vi "AddSingleOperation.vi"(6 "Timeout in ms (-1)":i32, 7 "At opposite end?":bool, 8 "error in (no error)":errorcluster, 10 "Operation":T1, 11 "SMP in":refnum<class "SMP.lvclass">) -> (0 "error out":errorcluster, 3 "SMP out":refnum<class "SMP.lvclass">)   [LabVIEW 2013, in "SMP.lvclass"]
doc: "Adds one individual operation, to the internal operations queue of the SMP object.\n\n<b>At opposite end?: </b>Set to TRUE to add the operation to the front of the internal operations queue. Default is FALSE.\n\n<b>Operations: </b>The operations to be added. Each operation has a name and data associated with it. Use this Data field to provide any data that the operation needs, except data produced by the operation which executes before it.\n\n<b>Timeout: </b>A timeout for the enqueue operation. Default is -1 (never time out)."
uses:
  SMP.lvclass
  Data types/operation.ctl
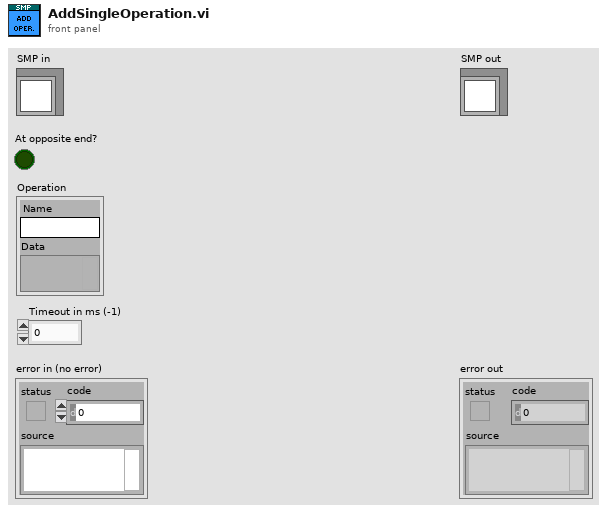
[diagram p1: front panel]
types:
  T1 = typedef "SMP.lvclass/operation.ctl" = cluster{"Name":string, "Data":variant}
  T2 = typedef "Pipe and Filter.lvclass/classData.ctl" = cluster{"Q ref":refnum<queue>, "Previous data":variant, "Current pipe":T3[]}
  T3 = typedef "Pipe and Filter.lvclass/operation.ctl" = cluster{"Name":string, "Data":variant}
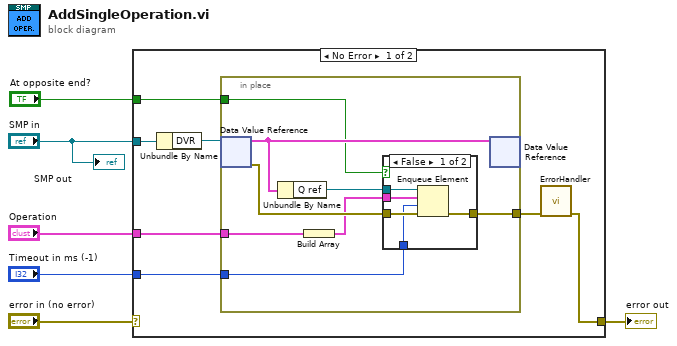
[diagram p0: block diagram]
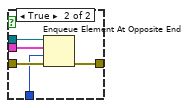
[diagram p2: hidden frame]
diagram:
  n1 = case shown="No Error" "error in (no error)" {
    selector: "error in (no error)" -> [_ w32]
    tunnel: [w9 w32] -> w5
    tunnel: "SMP in" -> [w12 _]
    tunnel: "Operation" -> [w11 _]
    tunnel: "At opposite end?" -> [w8 _]
    tunnel: "Timeout in ms (-1)" -> [w7 _]
    frame No Error {
      n2 = Unbundle By Name(w12) -> ("DVR"=w13:refnum<data-value>)
      n3 = in-place {
        in-place-border: w11 -> [w19]
        in-place-border: [w18] -> w10
        in-place-border: w8 -> [w15]
        in-place-border: w7 -> [w14]
        n4 = in-place-dvr #1(w13) -> (w21:T2, w17:errorcluster)
        n5 = Unbundle By Name(w21) -> ("Q ref"=w20:refnum<queue>)
        n6 = Build Array(w19) -> (w16:T1[])
        n7 = case shown="False" w15 {
          tunnel: w20 -> [w26 w31]
          tunnel: [w25 w30] -> w18
          tunnel: w17 -> [w24 w29]
          tunnel: w16 -> [w23 w28]
          tunnel: w14 -> [w22 w27]
          frame False {
            n8 = Enqueue Element(queue=w26, element=w23, timeout in ms (-1)=w22, error in (no error)=w24) -> (error out=w25:errorcluster)  [unwired: 2 out]
          }
          frame True {
            n9 = Enqueue Element At Opposite End(queue=w31, element=w28, timeout in ms (-1)=w27, error in (no error)=w29) -> (error out=w30:errorcluster)  [unwired: 2 out]
          }
        }
        n10 = in-place-dvr #1(w21) -> ()  [unwired: 2 out]
      }
      n11 = call "ErrorHandler.vi"("error in (no error)"=w10) -> ("error out"=w9:errorcluster)  [unwired: 9 in, 1 out]
    }
    frame Error {
    }
  }
  "error out" <- w5
  "SMP out" <- "SMP in"
